vi "DB_EscribeTablaVIF.vi"(8 "error in (no error)":errorcluster, 9 "VIF_cluster":T1, 10 "Equipo_Medicion":T2={"ID_EQUIPO"=0, "IP_EQUIPO"="", "NOMBRE_EQUIPO"="", "ESTADO_EQUIPO"="", "DESCRIPCION"="", "ID_MEDICION"=0, "ESTADO_MEDICION"="", "TIEMPO_MEDICION"="12-02-2019 18:41"}, 11 "db in":T3) -> (0 "error out":errorcluster, 3 "db out":T3)   [LabVIEW 2018]
uses:
  <vilib>/addons/database/Connection.llb/Conn ObjectReference.ctl
  Controls/Equipos_Medicion_cluster.ctl
  Controls/VIF_cluster.ctl
  <vilib>/addons/database/Connection.llb/Conn Execute.vi
  <vilib>/addons/database/Recordset.llb/Rec Destroy - Connection.vi
  <vilib>/addons/database/NI_Database_API.lvlib
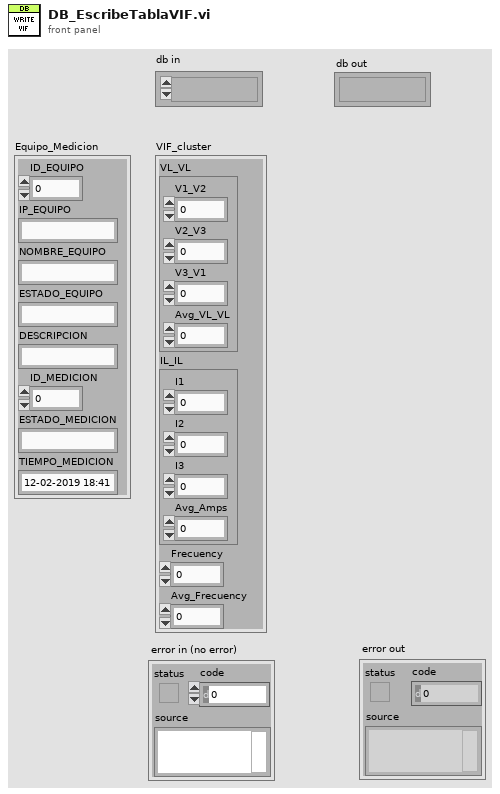
[diagram p1: front panel]
types:
  T1 = typedef "VIF_cluster.ctl" = cluster{"VL_VL":cluster{"V1_V2":sgl, "V2_V3":sgl, "V3_V1":sgl, "Avg_VL_VL":sgl}, "IL_IL":cluster{"I1":sgl, "I2":sgl, "I3":sgl, "Avg_Amps":sgl}, "Frecuency":sgl, "Avg_Frecuency":sgl}
  T2 = typedef "Equipos_Medicion_cluster.ctl" = cluster{"ID_EQUIPO":i32, "IP_EQUIPO":string, "NOMBRE_EQUIPO":string, "ESTADO_EQUIPO":string, "DESCRIPCION":string, "ID_MEDICION":i32, "ESTADO_MEDICION":string, "TIEMPO_MEDICION":string}
  T3 = typedef "NI_Database_API.lvlib/Conn ObjectReference.ctl" = refnum<k1>
  T4 = cluster{"V1_V2":sgl, "V2_V3":sgl, "V3_V1":sgl, "Avg_VL_VL":sgl}
  T5 = cluster{"I1":sgl, "I2":sgl, "I3":sgl, "Avg_Amps":sgl}
  T6 = typedef "NI_Database_API.lvlib/Rec ObjectReference.ctl" = refnum<k1>
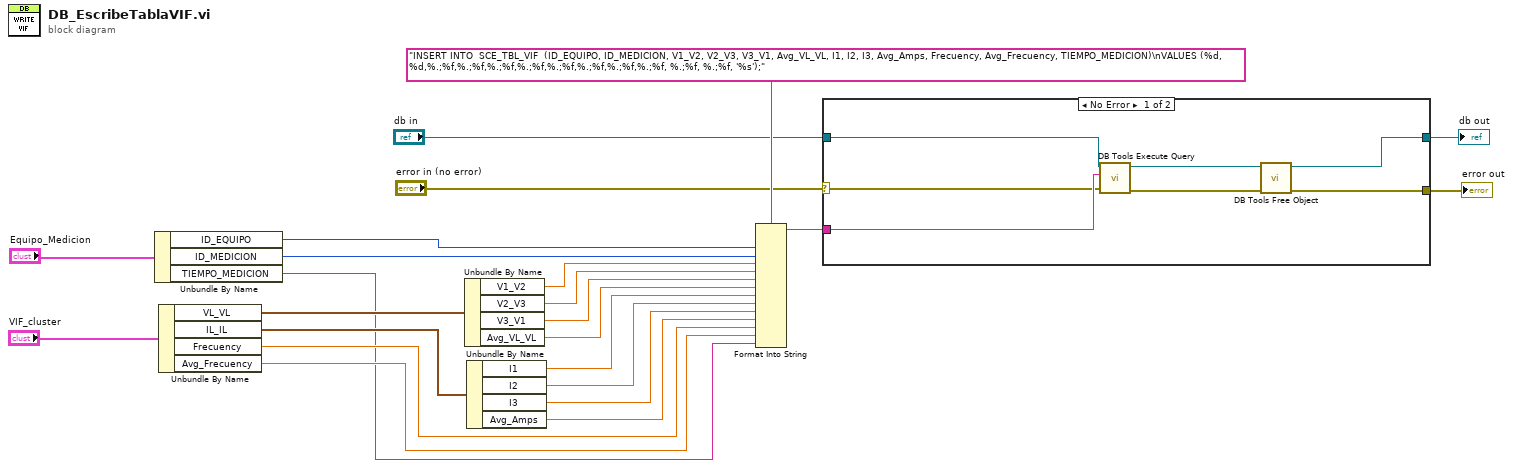
[diagram p0: block diagram]
diagram:
  n1 = Unbundle By Name("Equipo_Medicion") -> ("ID_EQUIPO"=w19:i32, "ID_MEDICION"=w18:i32, "TIEMPO_MEDICION"=w5:string)
  n2 = Unbundle By Name("VIF_cluster") -> ("VL_VL"=w12:T4, "IL_IL"=w11:T5, "Frecuency"=w7:sgl, "Avg_Frecuency"=w6:sgl)
  n3 = Unbundle By Name(w12) -> ("V1_V2"=w17:sgl, "V2_V3"=w16:sgl, "V3_V1"=w15:sgl, "Avg_VL_VL"=w10:sgl)
  n4 = Unbundle By Name(w11) -> ("I1"=w9:sgl, "I2"=w14:sgl, "I3"=w13:sgl, "Avg_Amps"=w8:sgl)
  n5 = Format Into String(format string="INSERT INTO  SCE_TBL_VIF  (ID_EQUIPO, ID_MEDICION, V1_V2, V2_V3, V3_V1, Avg_VL_VL, I1, I2, I3, Avg_Amps, Frecuency, Avg_Frecuency, TIEMPO_MEDICION)\nVALUES (%d, %d,%.;%f,%.;%f,%.;%f,%.;%f,%.;%f,%.;%f,%.;%f,%.;%f, %.;%f, %.;%f, '%s');" ("SQL"), w19, w18, w17, w16, w15, w10, w9, w14, w13, w8, w7, w6, w5) -> (resulting string=w23:string)  [unwired: 2 in, 1 out]
  n6 = case shown="No Error" "error in (no error)" {
    selector: "error in (no error)" -> [w28 w32]
    tunnel: w23 -> [w29 _]
    tunnel: [w26 w32] -> w21
    tunnel: "db in" -> [w27 w31]
    tunnel: [w24 w31] -> w3
    frame No Error {
      n7 = call-poly <vilib>:"DB Tools Execute Query.vi"("error in (no error)"=w28, "SQL query"=w29, "connection reference"=w27) -> ("error out"=w30:errorcluster, "recordset reference"=w25:T6)  [unwired: 5 in]
      n8 = call-poly <vilib>:"DB Tools Free Object.vi"("error in (no error)"=w30, "recordset reference"=w25) -> ("error out"=w26:errorcluster, "connection reference"=w24:T3)  [unwired: 8 in]
    }
    frame Error {
    }
  }
  "error out" <- w21
  "db out" <- w3
